vi "Demo_Read_Input_Command.vi"(8 "error in (no error)":errorcluster, 11 "CID IN":string="84F3EBBB070E") -> (0 "error out":errorcluster, 2 "JSON string":string, 3 "Topic":string)   [LabVIEW 2017]
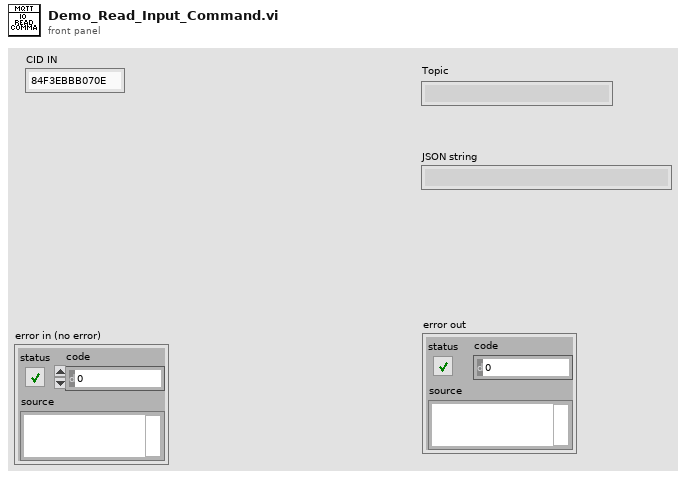
[diagram p1: front panel]
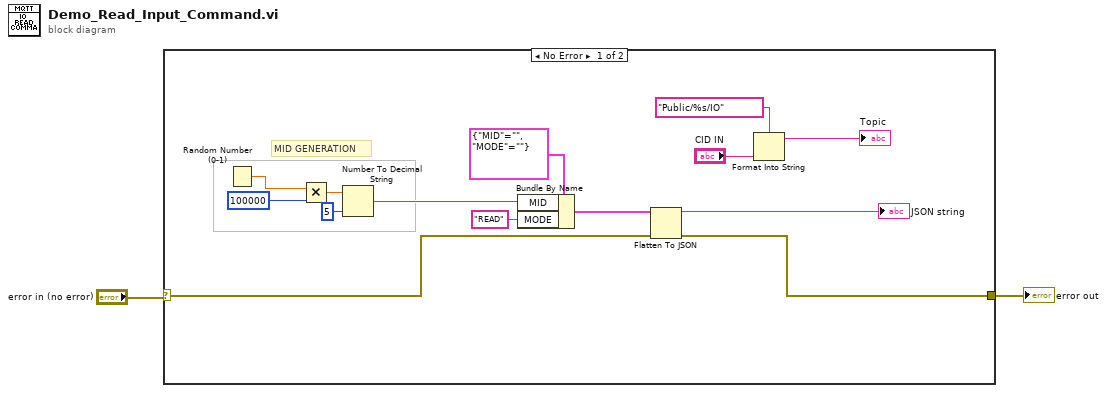
[diagram p0: block diagram]
diagram:
  n1 = case shown="No Error" "error in (no error)" {
    selector: "error in (no error)" -> [w6 w17]
    tunnel: [w7 w17] -> w2
    frame No Error {
      # "MID GENERATION"
      n2 = Random Number (0-1)() -> (number: 0 to 1=w15:dbl)
      n3 = Multiply(x=w15, y=100000) -> (x*y=w16:dbl)
      n4 = Number To Decimal String(number=w16, width (-)=i16 5) -> (decimal integer string=w12:string)
      n5 = Bundle By Name(cluster=cluster{"MID":string, "MODE":string} {"MID"="", "MODE"=""}, "MID"=w12, "MODE"="READ") -> (w9:cluster{"MID":string, "MODE":string})
      n6 = Flatten To JSON(anything=w9, error in (no error)=w6) -> (JSON string=→"JSON string":string, 11:w7:errorcluster)  [unwired: 1 in]
      n7 = Format Into String(format string="Public/%s/IO" ("Topic"), "CID IN") -> (resulting string=→"Topic":string)  [unwired: 2 in, 1 out]
    }
    frame Error {
    }
  }
  "error out" <- w2
